vi "IncrementShot.vi"(10 "Change":dbl, 11 "Shot":string) -> (2 "String":string, 3 "Numeric":i32)   [LabVIEW 2013]
doc: "Increments by 1 a shot string and returns the incremented shot as number and string."
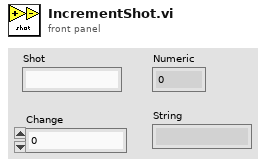
[diagram p1: front panel]
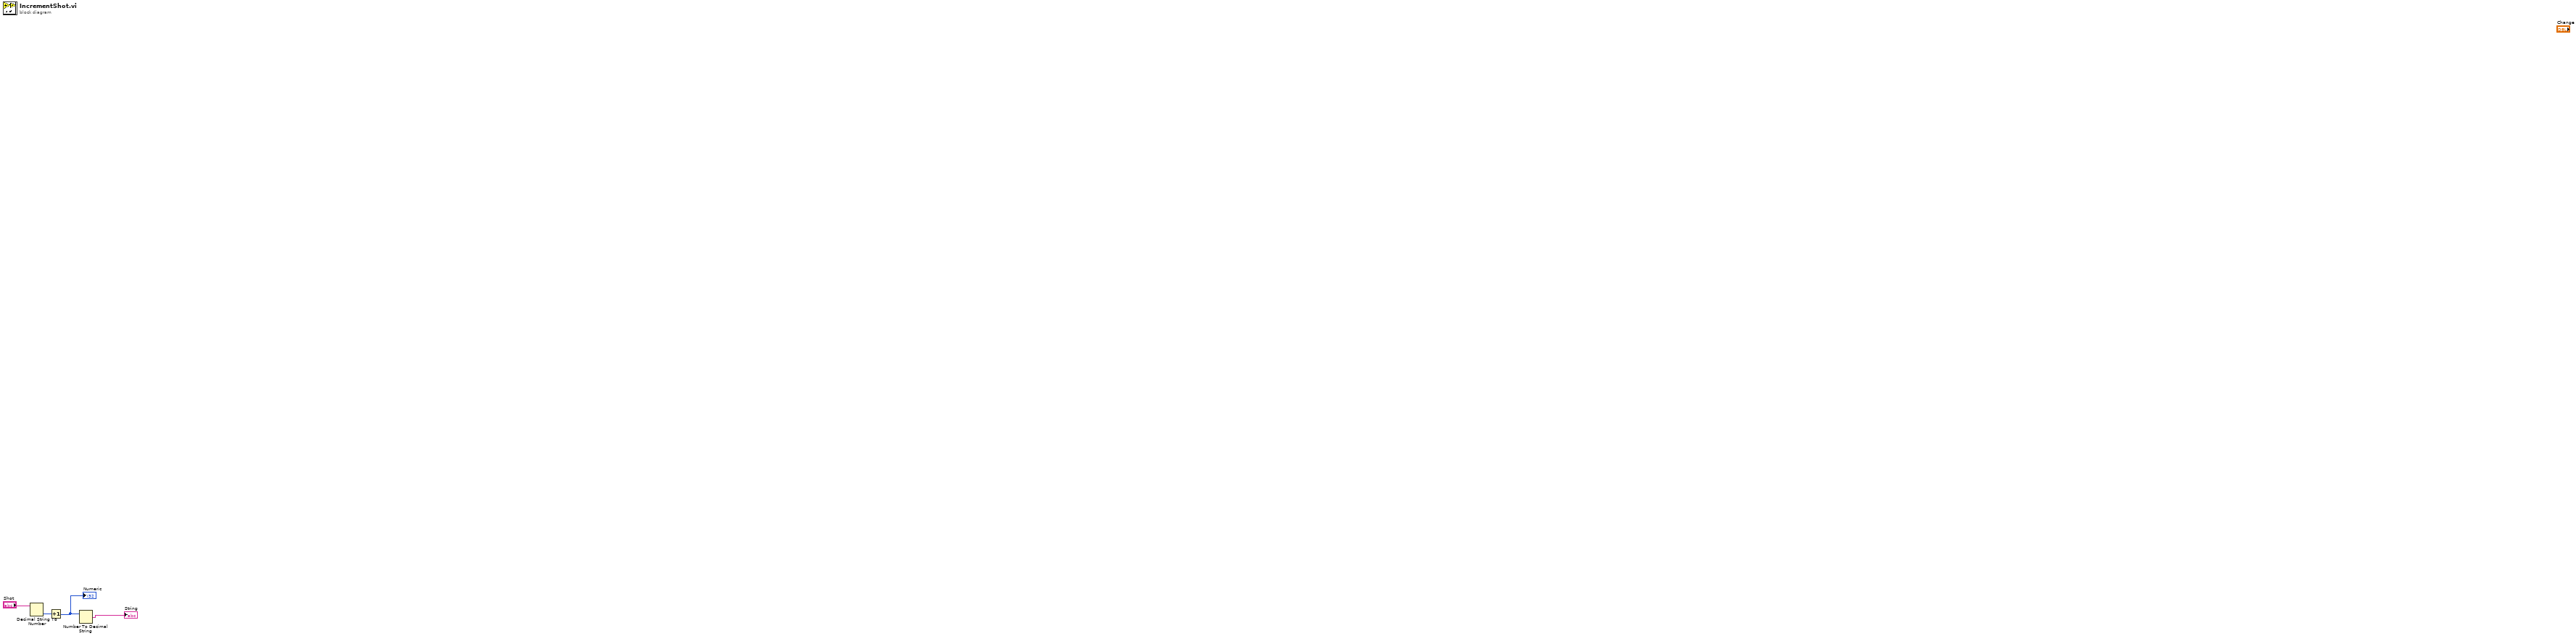
[diagram p0: block diagram]
diagram:
  n1 = Decimal String To Number(string="Shot") -> (number=w1:i32)  [unwired: 2 in, 1 out]
  n2 = Increment(x=w1) -> (x+1=w2:i32)
  "Numeric" <- w2
  n3 = Number To Decimal String(number=w2) -> (decimal integer string=→"String":string)  [unwired: 1 in]
